vi "Write_User_Answer.vi"(0 "Application_Directory":path, 7 "Data":string, 11 "Error_In":errorcluster, 13 "Key":string) -> (15 "Error_Out":errorcluster)   [LabVIEW 2023]
doc: "This VI Write Users Answer to INI files"
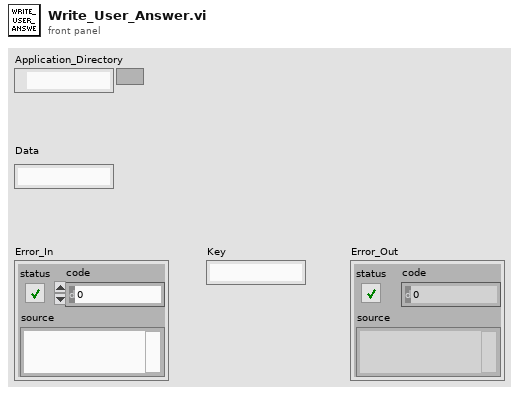
[diagram p1: front panel]
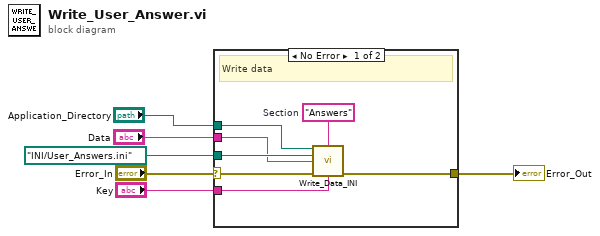
[diagram p0: block diagram]
diagram:
  n1 = case shown="No Error" "Error_In" {
    selector: "Error_In" -> [w10 w14]
    tunnel: "Application_Directory" -> [w13 _]
    tunnel: path "INI/User_Answers.ini" ("File_Name") -> [w12 _]
    tunnel: [w11 w14] -> w4
    tunnel: "Key" -> [w8 _]
    tunnel: "Data" -> [w7 _]
    frame No Error {
      w9 = "Answers"  # Section
      # "Write data"
      n2 = call "Write_Data_INI.vi"("Application_Directory"=w13, "Section"=w9, "File_Name"=w12, "Data"=w7, "Error_In"=w10, "Key"=w8) -> ("Error_Out"=w11:errorcluster)  [unwired: 8 in, 1 out]
    }
    frame Error {
    }
  }
  "Error_Out" <- w4
